vi "Get Control Ref Using Control Label.vi"(0 "reference in":refnum<class "Generic Utilities.lvclass">, 5 "error in (no error)":errorcluster, 7 "Control Label":string) -> (13 "Ref Found?":bool, 14 "reference out":refnum<class "Generic Utilities.lvclass">, 17 "Control Ref":refnum<vi>, 19 "error out":errorcluster)   [LabVIEW 2020, in "Generic Utilities.lvclass"]
uses:
  Generic Utilities.lvclass
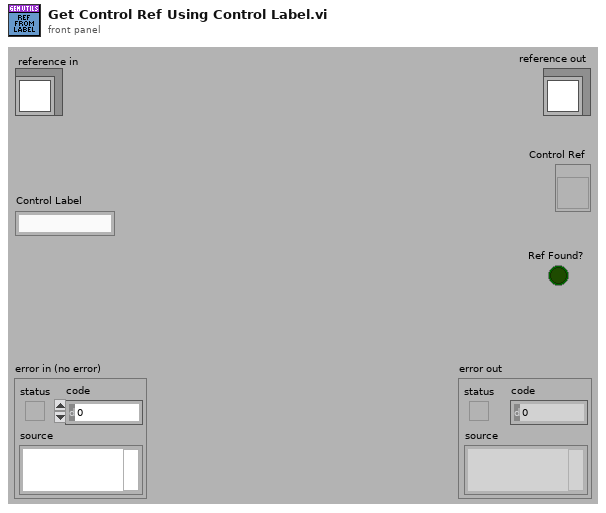
[diagram p1: front panel]
types:
  T1 = typedef "Generic Utilities.lvclass/ObjectAttributes.ctl" = cluster{"GUI Parameters":T2, "State Machine Control":cluster{"Timeout":i32, "State Queue":string[], "State History":string[], "State History Length":i32}, "Logging File Path":path, "OBJ not a refnum?":bool, "Timer Start":timestamp, "FP Refnums":T3}
  T2 = typedef "Generic Utilities.lvclass/GUI Parameters.ctl" = cluster{"Application Name":string, "GUI VI Ref":refnum<vi>, "Close Panel?":bool, "Message Window ref":refnum<vi>, "Version #":string}
  T3 = typedef "Generic Utilities.lvclass/FP Refnums.ctl" = cluster{"Panel refnum":refnum<vi>, "Control Labels":string[], "Refnums":refnum<vi>[]}
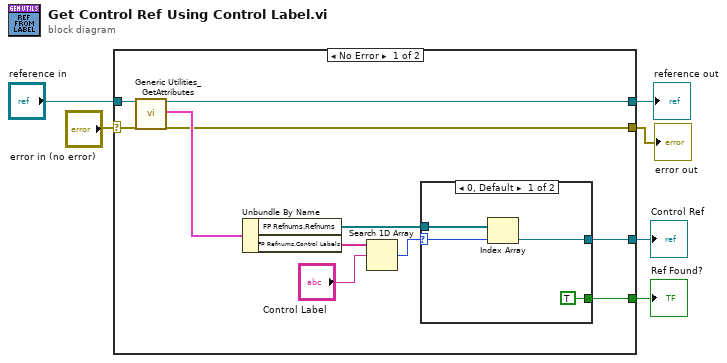
[diagram p0: block diagram]
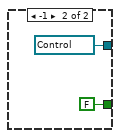
[diagram p2: hidden frame]
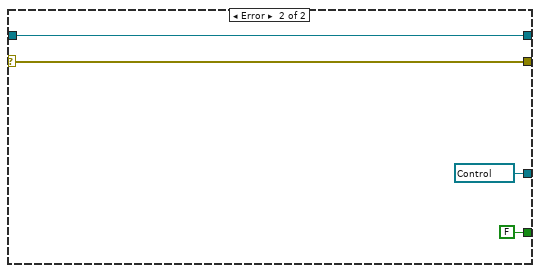
[diagram p3: hidden frame]
diagram:
  n1 = case shown="No Error" "error in (no error)" {
    selector: "error in (no error)" -> [w17 w27]
    tunnel: [w13 w27] -> w5
    tunnel: [w16 w26] -> w3
    tunnel: "reference in" -> [w14 w26]
    tunnel: [w8 refnum<vi> refnum ("Ctl Refnum")] -> w2
    tunnel: [w7 FALSE] -> w1
    frame No Error {
      n2 = call "Generic Utilities_GetAttributes.vi"("reference in"=w14, "error in (no error)"=w17) -> ("reference out"=w16:refnum<class "Generic Utilities.lvclass">, "attributes"=w15:T1, "error out"=w13:errorcluster)  [unwired: 14 in, 1 out]
      n3 = Unbundle By Name(w15) -> ("FP Refnums.Refnums"=w9:refnum<vi>[], "FP Refnums.Control Labels"=w12:string[])
      n4 = Search 1D Array(1D array=w12, element="Control Label") -> (index of element=w10:i32)  [unwired: 1 in]
      n5 = case shown="0, Default" w10 {
        selector: w10 -> [w20 _]
        tunnel: w9 -> [w21 _]
        tunnel: [w19 refnum<vi> refnum ("Ctl Refnum")] -> w8
        tunnel: [TRUE FALSE] -> w7
        frame 0, Default {
          n6 = Index Array(array=w21, index=w20) -> (element=w19:refnum<vi>)
        }
        frame -1 {
        }
      }
    }
    frame Error {
    }
  }
  "error out" <- w5
  "reference out" <- w3
  "Control Ref" <- w2
  "Ref Found?" <- w1
